vi "Version to String.vi"(11 "Version":T1) -> (3 "Version String":string)   [LabVIEW 2021, in "CIFCoreCommon.lvlib"]
uses:
  CIFCoreCommon.lvlib
  Typedef/Version Simple.ctl
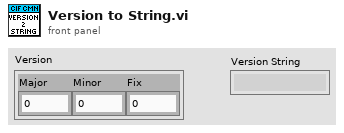
[diagram p1: front panel]
types:
  T1 = typedef "CIFCoreCommon.lvlib/Version Simple.ctl" = cluster{"Major":i32, "Minor":i32, "Fix":i32}
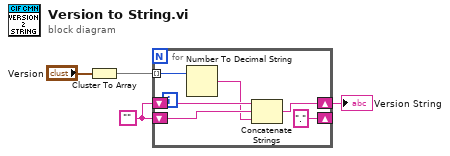
[diagram p0: block diagram]
diagram:
  w3 = ""
  n1 = Cluster To Array(cluster="Version") -> (array=w4:i32[])
  n2 = for {
    tunnel: w4 -> [w8] mode=indexing
    shift-right: ["."] -> _
    shift-left: w3 -> [w9]
    shift-right: [w6] -> w1
    shift-left: w3 -> [w10]
    n3 = Number To Decimal String(number=w8) -> (decimal integer string=w7:string)  [unwired: 1 in]
    n4 = Concatenate Strings(w10, w9, w7) -> (w6:string)
  }
  "Version String" <- w1
